vi "AlliGator Highlight Phasor ROI in Original Image v3.vi"(0 "AlliGator IV DVR in":refnum<data-value>, 1 "Image Color Scale Information":T2, 2 "Temp Overlay?":bool, 5 "Source Image Display":T1, 7 "Phasor Plot Image":T1, 9 "Phasor Plot ROI":T3, 11 "Error In":errorcluster, 12 "Overlay Color":u32(colorbox)) -> (4 "AlliGator IV DVR out":refnum<data-value>, 6 "Source Image Display out":T1, 8 "Phasor Plot Image Out":T1, 14 "CPU (s)":dbl, 15 "Error Out":errorcluster)   [LabVIEW 2021, in "AlliGator Source Image.lvlib"]
doc: "Compute and overlays the selected Phasor Plot ROI's pixels in the Source Image."
uses:
  AlliGator Source Image.lvlib
  Internal Variables/AlliGator Internal Variables v2.ctl
  <vilib>/vision/Image Controls.llb/IMAQ Image.ctl
  Internal Variables/AlliGator Gate Image Set.ctl
  Files/AlliGator FLI Dataset Type.ctl
  Files/AlliGator Data Series Type.ctl
  Dual-Channel Datasets/AlliGator Dataset Channel.ctl
  Settings/AlliGator Gate Arithmetic.ctl
  AlliGator Displayed Image.ctl
  Image/Named ROI Description.ctl
  Phasor Graph/AlliGator Decay Metadata v3.ctl
  Decay Analysis/Decay Preprocessing/AlliGator Decay Background Subtraction Info.ctl
  Decay Analysis/Decay Preprocessing/AlliGator Baseline Subtraction Method.ctl
  Graphs/XY Graph/XY Graph Plot Shift Parameters.ctl
  Graphs/XY Graph/XY Graph Plot Shift Method.ctl
  Decay Analysis/Decay Preprocessing/AlliGator Decay Extrapolation Parameters.ctl
  Phasor/Calibration Phasor (m, phi).ctl
  Phasor/Phasor Reference Series.ctl
  Phasor/Phasor Calibration Map v2.ctl
  Phasor/Phasor (g, s).ctl
  Phasor Graph/AlliGator Raw Phasor Plot Data v5.ctl
  Phasor/Phasor Standard Deviation Options.ctl
  Phasor Plot/AlliGator Phasor Multi-Harmonic Data.ctl
  Phasor/Phasor Harmonic Data.ctl
  Decay Fit Parameter Map/AlliGator Decay Fit Options & Parameters v4.ctl
  Fits/IRF(X)PSED/Decay Fit Options v4.ctl
  Fits/Decay Convolution/Decay Model.ctl
  Fits/Residual Type.ctl
  Fits/IRF(X)PSED/Fit Weights Type v2.ctl
  Fits/Non-linear Fitting Method v2.ctl
  Fits/Fit Calculation Method.ctl
  Fits/Non-linear Fitting Algorithm.ctl
  Decay Analysis/Decay Fit/AlliGator Decay Fit Parameter Constraints 2.ctl
  Fits/IRF(X)PSED/Decay Fit Parameters In List.ctl
  Fits/IRF(X)PSED/MLE Baseline Offset Type.ctl
  Decay Analysis/Decay Preprocessing/AlliGator Decay Preprocessing Parameters.ctl
  Fits/IRF(X)PSED/Decay Fit Parameters & Derived Quantities List v2.ctl
  Fits/IRF(X)PSED/Decay Fit Result Constraint.ctl
  Decay Fit Parameter Map/AlliGator Parameter Maps Data.ctl
  Image/Image Color Scale Information.ctl
  Globals, Variables, Constants/AlliGator Variables List.ctl
  Phasor Ratio/AlliGator Phasor Plot Reference Points.ctl
  ROIs/AlliGator ROI Manager Actions.ctl
  Palette/Image Palette Information.ctl
  Image/Image Display Palette Type.ctl
  Settings/AlliGator Settings List.ctl
  9cfa6bdc-d1e0-4e6c-94b8-050a3d16fc11.vi
  Variant/Variant to Data/Variant to Boolean.vi
  <vilib>/vision/NI_Vision_Development_Module.lvlib
  Globals, Variables, Constants/AlliGator Globals, Variables & Constants.lvlib
  Phasor Ratio/AlliGator Phasor Ratio.lvlib
  Error/Error.lvlib
  Settings/AlliGator Settings.lvlib
  Variant/Variant to Data/Variant to Data.lvlib
  Time/Time.lvlib
  ROIs/AlliGator ROIs.lvlib
  Utilities/Utilities.lvlib
  Image/Image.lvlib
  Palette/Palette.lvlib
  Phasor/Phasor.lvlib
  Decay Analysis/Decay Preprocessing/AlliGator Decay Preprocessing.lvlib
  Graphs/XY Graph/XY Graph Add-Ons.lvlib
  Phasor Graph/AlliGator Phasor Graph.lvlib
  Files/AlliGator Files.lvlib
  Phasor Plot/AlliGator Phasor Plot.lvlib
  Internal Variables/AlliGator Internal Variables.lvlib
  Fits/Fits.lvlib
  Decay Analysis/Decay Fit/AlliGator Decay Fit.lvlib
  Dual-Channel Datasets/AlliGator Dual-Channel Datasets.lvlib
  Decay Fit Parameter Map/AlliGator Decay Fit Parameter Map.lvlib
panel:
  in  "Image Color Scale":dbl(ramp)
  # "see the AlliGator License on the block diagram (Ctrl+E or Window:Show Block Diagram)"
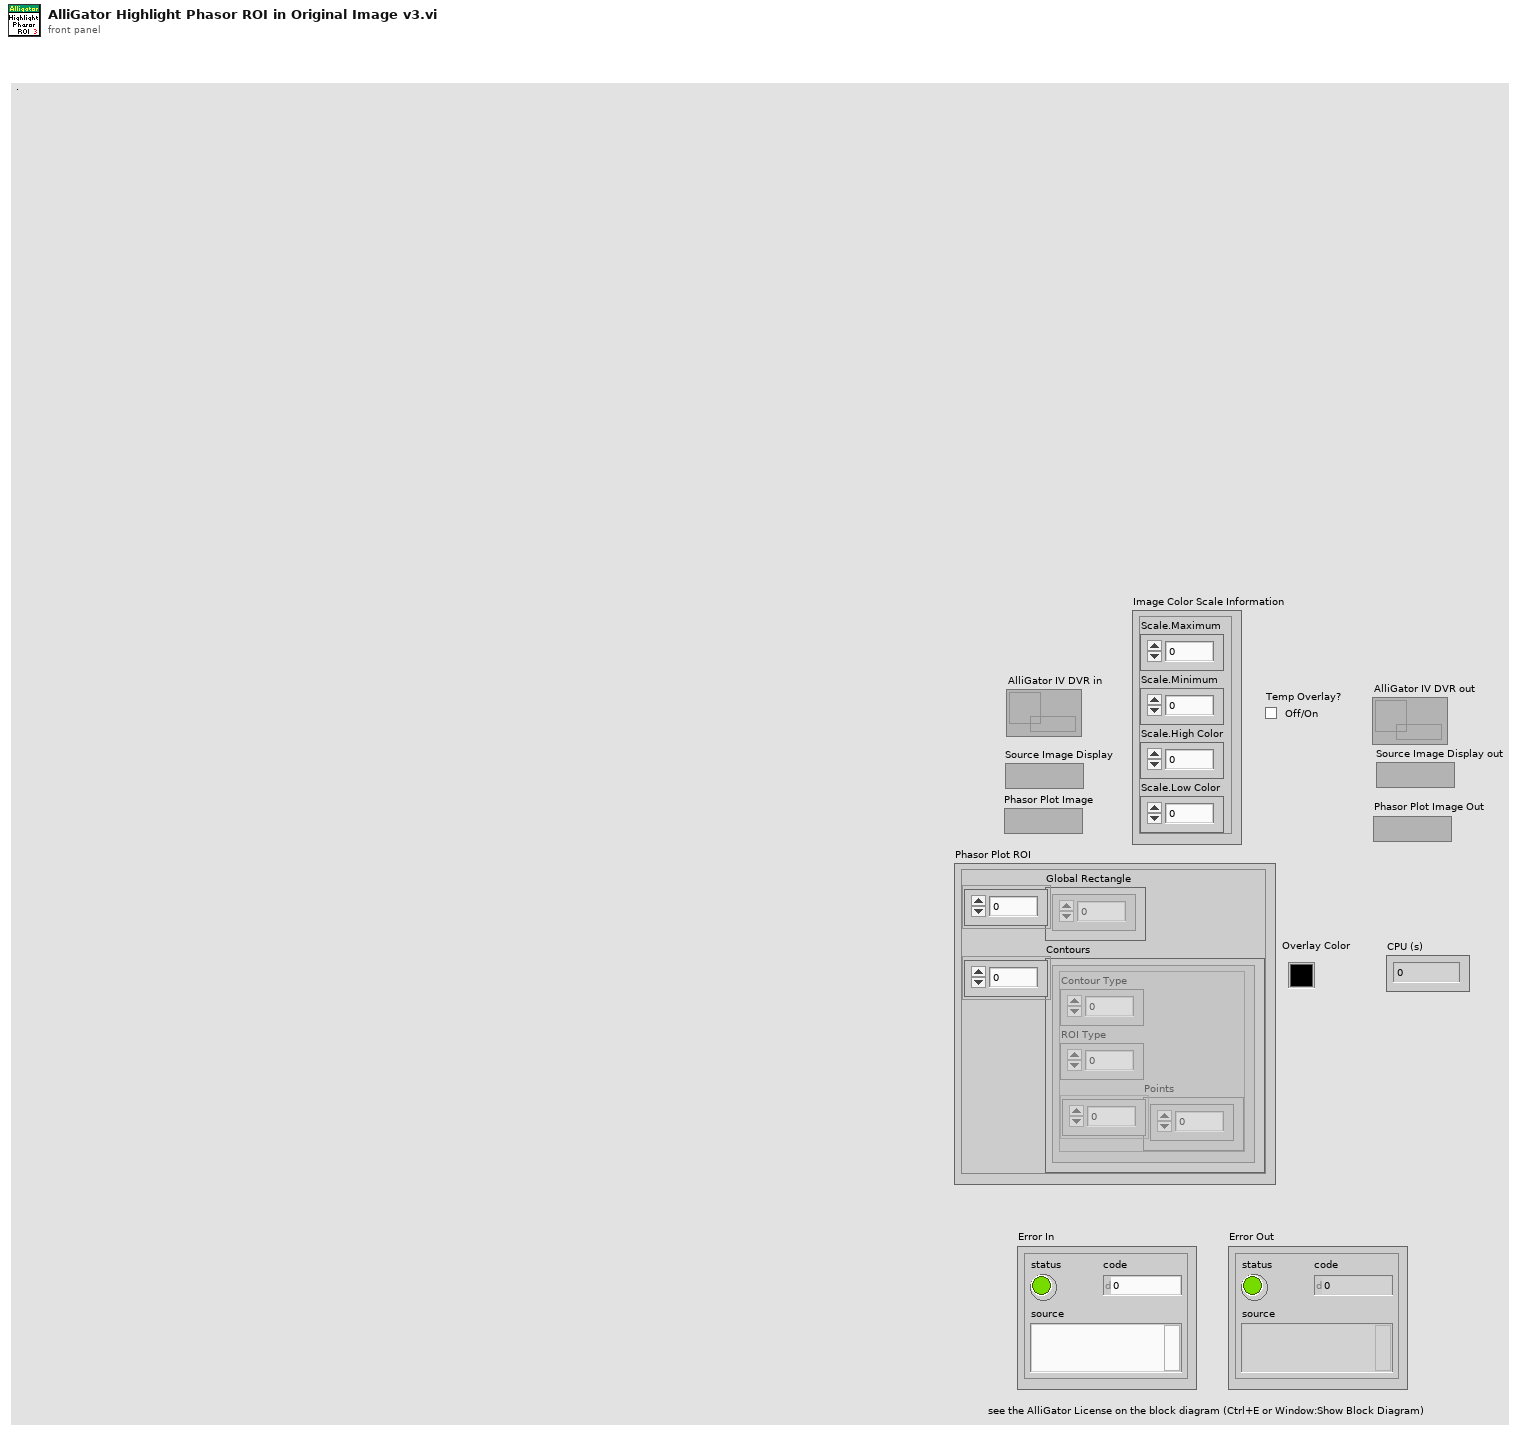
[diagram p1: front panel]
types:
  T1 = typedef "IMAQ Image.ctl" = refnum<image>
  T2 = typedef "Image.lvlib/Image Color Scale Information.ctl" = cluster{"Scale.Maximum":dbl, "Scale.Minimum":dbl, "Scale.High Color":u32, "Scale.Low Color":u32}
  T3 = cluster{"Global Rectangle":i32[], "Contours":cluster{"Contour Type":u32, "ROI Type":u32, "Points":i32[]}[]}
  T4 = typedef "AlliGator Settings.lvlib/AlliGator Settings List.ctl" = enum16{"GUI:Visible Settings Tab", "GUI:Last Run Version", "Source Image:Use Image Histogram for Contrast", "Source Image:Low Count Pixels Rejection Options", "Source Image:High Count Pixels Rejection Options", "Source Image:Use Image Brightness", "Source Image:Blend Overlay with Image Background", "Source Image:Use Fixed ROI Diameter", "Source Image:ROI Diameter", "Source Image:ROI Center Color", "Source Image:Peak Threshold", "Source Image:Intensity Threshold", "Source Image:Image Binning Options", "Source Image:Image Smoothing Options", "Source Image:Image Histogram Active", "Source Image:Invert Binary Mask", "Source Image:Hot Pixel Removal", "Source Image:Overlay Analyzed ROI Center", "Source Image:Auto-Adjust Contrast", "Source Image:Histogram Lower Percentile", "Source Image:Histogram Upper Percentile", "Source Image:Save Source Image", "Source Image:Scale Bar Options", "Source Image:Image Resolution (Pixel Size)", "Source Image:Flatfield Correction", "Source Image:Show Dead Left Columns Correction", "Source Image:Dead Left Columns Correction", "Source Image:Image Pre-Processing Operations Order", "Source Image:Overlay ROI Median", "Source Image:Median Overlay Color", "Data Information:Gate Width", "Data Information:Nanotime Gate Separation", "Data Information:Macrotime Gate Separation", "Data Information:Gate Step", "Data Information:# Gates", "Data Information:Gate Image Exposure", "Data Information:Gate Image Integration", "Data Information:Gates to Skip", "Data Information:Gates to Keep", "Data Information:Define Gates to", "Data Information:Channel Name", "Data Information:Available Channel Names", "Data Information:Channel Arithmetic", "Data Information:Background File Subtraction", "Data Information:Background File", "Data Information:Background Scaling Factor", "Data Information:Background Pile-up Correction", "Data Information:Background Pixel Well Capacity", "Data Information:Laser Period", "Data Information:SYNC Period", "Data Information:Pile-up Correction", "Data Information:Pixel Well Capacity", "Data Information:Dataset Scaling Factor", "Fluorescence Decay_Decay Pre-Processing:Reverse Gates", "Fluorescence Decay_Decay Pre-Processing:Verbose Decay Pre-Processing", "Fluorescence Decay_Decay Pre-Processing:Use Decay Pre-Processing", "Fluorescence Decay_Decay Pre-Processing:Background Subtraction", "Fluorescence Decay_Decay Pre-Processing:Background Definition Range", "Fluorescence Decay_Decay Pre-Processing:Baseline Subtraction Method", "Fluorescence Decay_Decay Pre-Processing:Decay Pre-Processing Operations Order", "Fluorescence Decay_Decay Pre-Processing:Smoothing Parameter", "Fluorescence Decay_Decay Pre-Processing:Shift Decay", "Fluorescence Decay_Decay Pre-Processing:Decay Shift Parameters", "Fluorescence Decay_Decay Pre-Processing:Fold Decay", "Fluorescence Decay_Decay Pre-Processing:# Folds", "Fluorescence Decay_Decay Pre-Processing:1-Normalize Decay", "Fluorescence Decay_Decay Pre-Processing:[0-1]-Normalize Decay", "Fluorescence Decay_Decay Pre-Processing:Smoothen Decay", "Fluorescence Decay_Decay Pre-Processing:Extrapolate Decay", "Fluorescence Decay_Decay Pre-Processing:Use Periodicity", "Fluorescence Decay_Decay Pre-Processing:Use Cursors", "Fluorescence Decay_Decay Pre-Processing:Tail Fraction", "Fluorescence Decay_Decay Pre-Processing:Head Fraction", "Fluorescence Decay_Decay Pre-Processing:Additional Points", "Fluorescence Decay_Decay Pre-Processing:Straighten Decay", "Fluorescence Decay_Decay Pre-Processing:Constant Background", "Fluorescence Decay_Decay Pre-Processing:Pixel-Normalize Decay", "Fluorescence Decay_Advanced Analysis:Extract IRF instead of Decay", "Fluorescence Decay_Advanced Analysis:IRF Extraction Options", "Fluorescence Decay_Advanced Analysis:IRF Optimization Options", "Fluorescence Decay_Advanced Analysis:Square Pulse Options", "Fluorescence Decay_Advanced Analysis:IRF Order", "Fluorescence Decay_Advanced Analysis:IRF Time Constants", "Fluorescence Decay_Advanced Analysis:Wavelet Analysis Options", "Fluorescence Decay_Advanced Analysis:Average Lifetime Options", "Fluorescence Decay_Fit Options:Fit Options", "Fluorescence Decay_Fit Options:Use Legacy Fitting Approach", "Fluorescence Decay_Fit Options:Use Data Information Laser Period", "Fluorescence Decay_Fit Parameters:Displayed Fit Parameters", "Fluorescence Decay_Fit Parameters:Fit Parameter Constraints", "Fluorescence Decay_Fit Parameters:Export Tabulated Results", "Fluorescence Decay_Fit Parameters:MLE Baseline Offset Type", "Fluorescence Decay_Fit Parameters:MLE Baseline Offset", "Fluorescence Decay_Fit Parameters:Guess Parameter Names", "Fluorescence Decay_Fit Parameters:Guess Parameter Values", "Fluorescence Decay_Fit Parameters:Guess Parameters Options", "Fluorescence Decay_Fit Parameters:Optimal Offset Selection Criterion", "Fluorescence Decay_Styles:Show Last Decay Only", "Fluorescence Decay_Styles:Decay Graph Color Array", "Fluorescence Decay:Decay Graph Active", "Fluorescence Decay Statistics:Min Peak Value", "Fluorescence Decay Statistics:Reject Low Decay Peak Pixels", "Fluorescence Decay Statistics:Reject High Decay Peak Pixels", "Fluorescence Decay Statistics:Max Peak Value", "Time Traces:Use File Timestamp", "Time Traces:Time Step", "Time Traces:Use Intensity Correction File", "Time Traces:Intensity Correction File", "Phasor Plot:Phasor Plot Smoothing Options", "Phasor Plot:Phasor Plot Size", "Phasor Plot:Phasor Plot Graphics Options", "Phasor Plot:Cumulative Phasor Plot", "Phasor Plot:Use Phasor Brightness", "Phasor Plot:Blend Overlay with Phasor Background", "Phasor Plot:Save Phasor Plot", "Phasor Plot:Show References", "Phasor Plot:Phasor Ratio Decay Range", "Phasor Plot:Exponential Fading", "Phasor Plot:Phasor Ratio Reference Colors", "Phasor Plot:Reference Radius", "Phasor Plot:Show Color Map Vertices", "Phasor Plot:Phasor Plot Active", "Phasor Plot:Phasor Ratio Color Map Type", "Phasor Plot:Phasor Ratio Color Map", "Phasor Plot:Phasor Ratio Display Range", "Phasor Plot:Selected Image ROI(s)", "Phasor Plot:All Image ROIs", "Phasor Plot:Selected Phasor Plot ROI(s)", "Phasor Plot:All Phasor Plot ROIs", "Phasor Plot:Phasor Ratio Color-Coded Quantity", "Phasor Plot:Store Phasor Harmonics", "Phasor Plot:Draw Reference Segment", "Phasor Plot:User-Defined Quantity", "Phasor Plot:Color Scale High Color", "Phasor Plot:Color Scale Low Color", "Phasor Plot:Intensity-weighted Phasor Plot", "Phasor Graph:Phasor Frequency", "Phasor Graph:Phasor Ratio Type", "Phasor Graph:Pixel-level Phasor Computation", "Phasor Graph:Save Phasor Graph", "Phasor Graph:Phasor Graph Active", "Phasor Graph:Phasor SDV Options", "Phasor Graph:Intensity-weighted Phasor Graph", "Phasor Graph:Define Shortest Lifetime as", "Phasor Calibration:Use Backup Calibration if needed", "Phasor Calibration:Backup Calibration Type", "Phasor Calibration:Calibration Type", "Phasor Calibration:Calibration Lifetime", "Phasor Calibration:Calibration Map Algorithm", "Single-Exponential Phasor Locus (SEPL):Gate Parameters", "Single-Exponential Phasor Locus (SEPL):User-defined Gate", "Single-Exponential Phasor Locus (SEPL):User-defined IRF", "Single-Exponential Phasor Locus (SEPL):Phasor Parameters", "Single-Exponential Phasor Locus (SEPL):Decay & IRF Parameters", "Single-Exponential Phasor Locus (SEPL):Display Parameters", "Lifetime Analysis:Decay Analysis Parameters", "Lifetime Analysis:Lifetime Map Active", "Plugins:Python Settings", "Miscellaneous:Verbose Mode", "Miscellaneous:Beep after Script", "Miscellaneous:Saved Image File Format", "Miscellaneous:Exported Gate Image Settings", "Miscellaneous:Include Loading in Timing", "Miscellaneous:Verbose Settings Mode", "Miscellaneous:Histogram Options", "Miscellaneous:Beep on Error", "Miscellaneous:# Logical Processors Used", "Miscellaneous:ROI Description Max Characters", "Miscellaneous:Verbose Error Mode", "Miscellaneous:Transparent Mask Color"}
  T5 = typedef "Palette.lvlib/Image Palette Information.ctl" = cluster{"Palette Name [# Colors,int?,inv?]":string, "Palette Type":T6, "Palette Colors":u32[], "Interpolate?":bool}
  T6 = typedef "Image.lvlib/Image Display Palette Type.ctl" = u32
  T7 = typedef "AlliGator Globals, Variables & Constants.lvlib/AlliGator Variables List.ctl" = enum16{"---- GUI ----", "GUI:Initialization Status", "GUI:State Indicators Refnum", "GUI:Original AlliGator Menu Items", "GUI:Current Action Loop State", "GUI:Script in progress", "GUI:Playback", "GUI:Loop Playback", "GUI:Search ROI Used", "GUI:Search ROI", "Decay Graph Max Legend Size", "Intensity Graph Max Legend Size", "Decay Statistics Graph Max Legend Size", "Phasor Graph Max Legend Size", "Phasor Ratio Graph Max Legend Size", "Lifetime Graph Max Legend Size", "---- Files ----", "Files:Export Dataset Frames as Individual Files", "Files:Show Batch Export Help Balloons", "Files:Frames in Dataset", "Files:ptu File Frame Start Indices", "Files:Current Frame in Dataset", "Files:Current Frame Timestamp", "Files:Dataset Loaded", "Files:Dataset Metadata", "Files:Dataset Channel", "Files:Dataset Data Description", "Files:Background Dataset Metadata", "Files:Background Dataset Channel", "Files:Background Dataset Data Description", "Files:Background File Subtraction", "Files:Background File Path", "Files:Background File Pile-up Correction", "Files:Background File Pixel Well Capacity", "Files:Background File Scaling Factor", "Files:Current Dataset Load Settings", "Files:Dataset Path", "Files:ICCD-specific Information", "Files:Macrotime Gate Separation", "------ Python Plugins ------", "Python Plugins:Information", "Python Plugins:Python Session", "Python Plugins:Valid Python Session?", "---- Source Image ----", "Source Image:ROIs", "Source Image:Current ROI", "Source Image:ROI Event Refnum", "X_Source Image:Display Range", "X_Source Image:Palette Information", "X_Source Image:Type of Displayed Image", "X_Time Gate Slider", "Source Image:Palette List", "Source Image:Scale", "Source Image:ROI Overlay Color", "Source Image:Overlay to Erase", "Source Image:Is Displayed Image Accumulated", "Source Image:White Light Image Modified", "Source Image:Mask Image Modified", "---- Image Profile Window ----", "Image Profile:Window Event Refnum", "Image Profile:IntensityType", "Image Profile:Intensity Average Type", "Image Profile:Intensity-weighted SDV", "Image Profile:Box Profile Type", "Image Profile:Window Open", "Image Profile:Plotted Fit Parameter", "------ Phasor Graph -------", "Phasor Graph:Show Line", "---- Phasor Plot ---", "Phasor Plot:Parameters Changed", "Phasor Plot:FLI Dataset Modified since last Calculation", "Phasor Harmonics Data", "Selected Phasor Harmonics", "Phasor Harmonic Manager Event Refnum", "Phasor Plot:ROIs", "Phasor Plot:Current ROI", "Phasor Plot:ROI Event Refnum", "Phasor Plot:Image Reference Points", "Phasor Plot:Computed", "Phasor Plot:Palette Information", "Phasor Plot:Palette List", "Phasor Plot:Phasor Ratio Palette Information", "Phasor Plot:Phasor Ratio Palette List", "Phasor Plot:Image Scale", "Phasor Plot:Image Overlay to Erase", "Phasor Plot:Image Elements to Update", "Phasor Plot:Current Calculation Parameters", "Phasor Plot:Current Calibration Options", "Phasor Plot:Reset Cumulated Phasor Plot", "Phasor Plot:Reference 1", "Phasor Plot:Lifetime Reference 1", "Phasor Plot:Reference 1 Frequency", "Phasor Plot:Reference 2", "Phasor Plot:Lifetime Reference 2", "Phasor Plot:Reference 2 Frequency", "---- Decay Analysis ----", "Number of Selected Decays to Fit", "LS Fit Results", "LAR Fit Results", "BS Fit Results", "Last Decay Max - Min", "Best Fit Parameters", "Best Fit Parameter Names", "Actual Size X", "Actual Size Y", "Binning X", "Binning Y", "Actual # Gates", "Dataset Number", "Gates to...", "Gates Skipped", "Gates to keep", "Gate Step", "Gate Separation", "Reversed Gates", "Pile-up Correction", "Pixel Well Capacity", "Background Subtracted", "Background Subtraction Method", "Background Definition Range", "Background File (deprecated)", "Number of Dataset Accumulated", "Array of Accumulated Dataset Paths", "Do Averaged Datasets", "Destination File Path", "Process Plot Target", "Use 1/D as Phasor Frequency", "---- Decay Fit Parameter Map -----", "Decay Fit Parameter Map:Palette Information", "Decay Fit Parameter Map:Palette List", "Decay Fit Parameter Map:X Resolution", "Decay Fit Parameter Map:Y Resolution", "Decay Fit Parameter Map:Use Decay Fit Result Constraints", "Decay Fit Parameter Map:Decay Fit Result Constraints", "Decay Fit Parameter Map:Decay Fit Result Constraints Applied", "---- Parameter Map ----", "Parameter Map:Palette Information", "Parameter Map:Palette List", "------- Local Decay Window ---------", "Local Decay Graph Window:Event Refnum", "Local Decay Graph Window:Use normalized IRF for convolution", "----- Miscellaneous ----", "Misc:Skippable Dialog Windows Status"}
  T8 = typedef "AlliGator ROIs.lvlib/AlliGator ROI Manager Actions.ctl" = enum16{"Undefined", "Delete Current ROI", "Delete All Unselected ROIs", "Delete Multiple ROIs", "Delete All ROIs", "Swap ROIs", "Insert ROI", "Update Current ROI Descriptor", "Rename Current ROI", "Store New ROI", "Store Multiple ROIs", "Select Next ROI", "Select Previous ROI", "Find Selected ROI", "Show All ROIs", "Update ROI Manager Window", "Merge All ROIs", "Unmerge ROI", "Set Selected ROI by ID"}
  T9 = typedef "AlliGator Phasor Ratio.lvlib/AlliGator Phasor Plot Reference Points.ctl" = cluster{"O_h":dbl, "O_v":dbl, "1_h":dbl, "1_v":dbl}
  T10 = typedef "AlliGator Internal Variables.lvlib/AlliGator Internal Variables v2.ctl" = cluster{"----------------------------- Images -----------------------------":u8, "Displayed Image":T1, "White Light Image":T1, "Mask Image":T1, "ROI Mask Image":T1, "Current Dataset Images 1":T11, "Background Dataset Images 1":T11, "Current Dataset Images 2":T11, "Background Dataset Images 2":T11, "Current Dataset Arithmetic Images":T11, "Accumulated Dataset Images 1":T11, "Accumulated Dataset Images 2":T11, "Accumulated Dataset Arithmetic Images":T11, "----------------------------- File Paths -----------------------------":u8, "Phasor Plot Image":T1, "Decay Fit Parameter Map Image":T1, "Parameter Map Image":T1, "Single Data Point Path":path, "White Light Image Path":path, "Mask Image Path":path, "Time-Series Folder":path, "[Time-Series Paths]":path[], "----------------------------- FLI Dataset -----------------------------":u8, "Current Dataset":i32, "Single Dataset Type":T12, "Current Folder":string, "AlliGator Data Series Type":T13, "# Datasets":i32, "Dual-Channel Dataset":bool, "Selected Channel Name":string, "Dataset Channel":T14, "Channel Arithmetic":T15, "Dual-Channel Background Dataset":bool, "Background Channel":T14, "Dual-Channel Accumulated Dataset":bool, "Start Time":dbl, "[Time-Series Timestamps]":dbl[], "[Intensity Corrections]":dbl[], "Time Series Script":bool, "Type of Displayed Image":T16, "Gate Image Slide":u16, "# Gates":i32, "ROIs":T17[], "----------------------------- Decays -----------------------------":u8, "ROI Decay":cluster{"t Array":dbl[], "I Array":dbl[]}, "Valid Decay":bool, "Decay  Metadata":T19, "Reference Decay Plot Name":string, "Reference Decay":cluster{"t Array":dbl[], "I Array":dbl[]}, "Decay Shift Plot":cluster{"Time Stamps":dbl[], "Decay Shifts":dbl[]}, "[Decays Max Values]":sgl[], "[Decays Min Values]":sgl[], "----------------------------- Calibration -----------------------------":u8, "Calibration Phasor":T25, "Calibration Phasor Series":T26, "Phasor Calibration Map":T27, "Calibration Map MD5 Digest":string, "----------------------------- Phasor Graph -----------------------------":u8, "Last Raw Phasor":T28, "Last Calibrated Phasor":T28, "Last Calibrated Phasor SDV":T28, "Phasor Graph:Phasor Plot":cluster{"g Array":dbl[], "s Array":dbl[]}, "Phasor Graph:Phasor SDV Plot":cluster{"g Array":dbl[], "s Array":dbl[]}, "[Phasor Graph:Raw Phasor Plots]":T29[], "Phasor Plot locked to Ref 1":i32, "[Phasor Plot(s) locked to Ref 1]":i32[], "[Phasor Plot(s) locked to Ref 2]":i32[], "[Pixel Phasors]":T28[], "----------------------------- Phasor Plot -----------------------------":u8, "[[Sum Image]]":dbl[][], "[[CSG Phasors]]":csg[][], "[[Valid Pixel?]]":bool[][], "[[Phasor Ratios]]":dbl[][], "[[Average Lifetimes]]":dbl[][], "Amplitude Weighted Average Lifetime":bool, "I/m/phi Dataset":cluster{"I/m/phi Dataset?":bool, "Base Frequency":dbl[unit], "Harmonic Orders":u8[]}, "Multi Phasor Plot Data":T31, "----------------------------- Decay Fit Parameter Map -----------------------------":u8, "Decay Fit Options & Parameters":T33, "Fit Options: Decay Preprocessing Parameters":T44, "Fit Options: Reference Decay":cluster{"t Array":dbl[], "I Array":dbl[]}, "Is Full Image Parameters Map":bool, "Is Single-Pixels Parameters Map":bool, "NLSF Parameters Map X Resolution":i32, "NLSF Parameters Map Y Resolution":i32, "[Single Decay Fit Parameters]":dbl[], "Fit Model":T35, "[[Multiple Decays Fit Parameters]]":dbl[][], "[[Multiple Decays Fit Parameter SDVs]]":dbl[][], "[[IRFs]]":dbl[][], "[ROI Descriptors]":T18[], "IRF Array Time Axis":dbl[], "Decay Array Time Axis":dbl[], "[Decay Fit Parameter Names]":T45[], "[Decay Sum]":dbl[], "Array of Decay Fit Result Constraints":T46[], "Selected ROIs Array":bool[], "----------------------------- Parameter Maps -----------------------------":u8, "[Map Set Names]":string[], "[Parameter Maps]":T47[], "[[User-defined Quantities]]":dbl[][], "User-defined Quantity":string}
  T11 = typedef "AlliGator Internal Variables.lvlib/AlliGator Gate Image Set.ctl" = cluster{"SGL Gate Images":T1[], "SGL Sum Image":T1, "SGL Max Image":T1, "SGL Min Image":T1}
  T12 = typedef "AlliGator Files.lvlib/AlliGator FLI Dataset Type.ctl" = enum16{"HDF5 FLI Dataset", "Gate Image Folder", ".sdt FLI Dataset (Becker & Hickl)", ".ptu FLI Dataset (PicoQuant)", "SS1 FLI Dataset", "SS2 FLI Dataset", "I/m/phi Dataset", ".bin FLI Dataset (PicoQuant Binned)", ".bin FLI Dataset (Piccolo Binned)", ".mat FLI Dataset"}
  T13 = typedef "AlliGator Files.lvlib/AlliGator Data Series Type.ctl" = enum16{"Not a Supported Series", "Gate Images Folder Series", "SwissSPAD 2 Dataset Series", "B&H FLI Dataset Series", "PicoQuant PTU FLI Dataset Series", "PicoQuant BIN FLI Dataset Series", "Piccolo hist BIN FLI Dataset Series", "HDF5 FLI Dataset Series"}
  T14 = typedef "AlliGator Dual-Channel Datasets.lvlib/AlliGator Dataset Channel.ctl" = enum16{"G2", "INT"}
  T15 = typedef "AlliGator Settings.lvlib/AlliGator Gate Arithmetic.ctl" = enum16{"None", "INT-G2", "G2/INT*<INT>", "(1 - G2/INT)*<INT>"}
  T16 = typedef "AlliGator Source Image.lvlib/AlliGator Displayed Image.ctl" = enum16{"Single Gate", "Sum of All Gates", "Max of All Gates", "Min of All Gates", "-", "White Ligth Image", "Mask Image"}
  T17 = typedef "Image.lvlib/Named ROI Description.ctl" = cluster{"ROI Descriptor":T18, "ROI Name":string, "Overlay Color":u32}
  T18 = typedef "ROI Descriptor" = cluster{"Global Rectangle":i32[], "Contours":cluster{"ID":enum32{"External", "Internal"}, "Type":u32, "Coordinates":i32[]}[]}
  T19 = typedef "AlliGator Phasor Graph.lvlib/AlliGator Decay Metadata v3.ctl" = cluster{"ROI Descriptor":T18, "ROI Center":cluster{"X":i32, "Y":i32}, "Decay Background Subtraction Info":T20, "Decay Reverted":bool, "Decay Smoothened":bool, "Decay Straightened":bool, "Fitted Tau (Decay Straightening)":dbl, "Decay Shift Parameters":T22, "Decay Shifted":bool, "Decay Extrapolated":bool, "Decay Extrapolation Parameters":T24, "Decay Normalized":bool, "Fold Decay":bool, "# Folds":u32}
  T20 = typedef "AlliGator Decay Preprocessing.lvlib/AlliGator Decay Background Subtraction Info.ctl" = cluster{"Laser Period":dbl[unit], "Gate Duration":dbl[unit], "Baseline Subtraction Method":T21, "Background Definition Range":cluster{"Min Gate":dbl[unit], "Max Gate":dbl[unit]}, "Total Intensity w/o Bkgd Subtraction":dbl, "Bkgd-subtracted Intensity (exp)":dbl, "# Data Points":i32, "Background/Gate":dbl, "Fitted Lifetime":dbl[unit], "Bkgd-subtracted Intensity (theo)":dbl}
  T21 = typedef "AlliGator Decay Preprocessing.lvlib/AlliGator Baseline Subtraction Method.ctl" = enum16{"Mean", "Min", "Square Gated Single-Exponential", "File", "Constant"}
  T22 = typedef "XY Graph Add-Ons.lvlib/XY Graph Plot Shift Parameters.ctl" = cluster{"Type":T23, "Shift":dbl[unit], "Threshold":dbl, "Rotate":bool}
  T23 = typedef "XY Graph Add-Ons.lvlib/XY Graph Plot Shift Method.ctl" = enum16{"Default", "CFD", "Threshold", "Cross-Correlation"}
  T24 = typedef "AlliGator Decay Preprocessing.lvlib/AlliGator Decay Extrapolation Parameters.ctl" = cluster{"Additional Points":u32, "Head Fraction":dbl, "Fitted Tau":dbl, "Use Periodicity":bool, "Use Cursors":bool, "Tail Fraction":dbl}
  T25 = typedef "Phasor.lvlib/Calibration Phasor (m, phi).ctl" = cluster{"m":dbl, "phi":dbl, "Phasor Frequency":dbl[unit], "Reference Lifetime":dbl[unit]}
  T26 = typedef "Phasor.lvlib/Phasor Reference Series.ctl" = cluster{"m Array":dbl[], "phi Array":dbl[], "Phasor Frequency":dbl[unit], "Calibration Lifetime":dbl[unit]}
  T27 = typedef "Phasor.lvlib/Phasor Calibration Map v2.ctl" = cluster{"Phasor Frequency":dbl[unit], "Calibration Lifetime":dbl[unit], "ROI Centers":cluster{"X":i32, "Y":i32}[], "ROI Descriptors":T18[], "Map Resolution X":i32, "Map Resolution Y":i32, "z Array":cdb[]}
  T28 = typedef "Phasor.lvlib/Phasor (g, s).ctl" = cluster{"g":dbl, "s":dbl}
  T29 = typedef "AlliGator Phasor Graph.lvlib/AlliGator Raw Phasor Plot Data v5.ctl" = cluster{"Phasor Plot Name":string, "Raw Phasor Plot":T28[], "Phasor Frequency":dbl[unit], "[Decay Metadata]":T19[], "Raw Phasor Plot SDV":T28[], "Phasor SDV Options":T30, "[Calibration Phasor]":T25[], "Intensity Array":dbl[]}
  T30 = typedef "Phasor.lvlib/Phasor Standard Deviation Options.ctl" = cluster{"Compute Estimated SDV":bool, "# Replicas":u32, "Use Estimated Average Phasor":bool}
  T31 = typedef "AlliGator Phasor Plot.lvlib/AlliGator Phasor Multi-Harmonic Data.ctl" = cluster{"Base Frequency":dbl[unit], "# Harmonics":u8, "Harmonic Orders":u8[], "Phasor Plot Settings Checksum":u64, "Phasor Harmonic Data Array":T32[]}
  T32 = typedef "Phasor.lvlib/Phasor Harmonic Data.ctl" = cluster{"Phasor Harmonic Name":string, "Phasor Plot Settings Checksum":u64, "Phasor Frequency":dbl[unit], "Base Frequency":dbl[unit], "Harmonic Order":u8, "Phasor Plot Parameters":string, "Phasor Array [[CSG]]":csg[][], "Dataset File Path":path}
  T33 = typedef "AlliGator Decay Fit Parameter Map.lvlib/AlliGator Decay Fit Options & Parameters v4.ctl" = cluster{"SYNC Period":dbl[unit], "Fit Options":T34, "Fit Parameter Constraints":T41[], "MLE Baseline Offset":dbl, "MLE Baseline Offset Type":T43}
  T34 = typedef "Fits.lvlib/Decay Fit Options v4.ctl" = cluster{"Show Fit Residuals":bool, "Fit Model":T35, "Residual Type":T36, "Max Decay Percentile":dbl, "Min Decay Percentile":dbl, "Show Full Decay":bool, "Weights":T37, "Fitting Method":T38, "Compute Parameter Uncertainties":bool, "Periodic Boundaries":bool, "Model Calculation":T39, "Period":dbl[unit], "Termination Criteria":cluster{"Max Iterations":i32, "Max Function Calls":i32, "Max Time":dbl[unit], "Function Tolerance":dbl, "Parameter Tolerance":dbl, "Gradient Tolerance":dbl, "Min Lambda":dbl, "Max Lambda":dbl, "Initial Tick Count":u32}, "Offset Resolution":dbl[unit], "Use Local IRF":bool, "Fitting Algorithm":T40, "Show Confidence Interval ":bool, "Confidence Level":dbl}
  T35 = typedef "Fits.lvlib/Decay Model.ctl" = enum16{"1-Exponential", "2-Exponentials"}
  T36 = typedef "Fits.lvlib/Residual Type.ctl" = enum16{"Standard", "Normalized", "Reduced"}
  T37 = typedef "Fits.lvlib/Fit Weights Type v2.ctl" = enum16{"Unweighted", "1/Variance (Neyman)", "1/Variance (Pearson)", "Best of All"}
  T38 = typedef "Fits.lvlib/Non-linear Fitting Method v2.ctl" = enum16{"Least Square", "Least Absolute Residual", "Bisquare", "MLE", "-", "Best of All"}
  T39 = typedef "Fits.lvlib/Fit Calculation Method.ctl" = enum16{"Simulation", "Convolution", "Integration"}
  T40 = typedef "Fits.lvlib/Non-linear Fitting Algorithm.ctl" = enum16{"Levenberg-Marquardt", "Trust-Region Dogleg"}
  T41 = typedef "AlliGator Decay Fit.lvlib/AlliGator Decay Fit Parameter Constraints 2.ctl" = cluster{"Fit Parameter":T42, "Min Value":dbl, "Max Value":dbl, "Global":bool, "Used":bool}
  T42 = typedef "Fits.lvlib/Decay Fit Parameters In List.ctl" = enum16{"Offset", "Baseline", "A_1", "tau_1", "A_2", "tau_2"}
  T43 = typedef "Fits.lvlib/MLE Baseline Offset Type.ctl" = enum32{"Absolute", "Percentage"}
  T44 = typedef "AlliGator Decay Preprocessing.lvlib/AlliGator Decay Preprocessing Parameters.ctl" = cluster{"Background Subtraction":bool, "Straighten Decay":bool, "Reverse Gates":bool, "1-Normalized Decay":bool, "Smoothen Decay":bool, "Smoothing Parameter":dbl, "Shift Decay":bool, "Decay Shift Parameters":T22, "Extrapolate Decay":bool, "Additional Points":u32, "Head Fraction":dbl, "Pixel-Normalize Decay":bool, "Use Periodicity":bool, "Use Cursors":bool, "Tail Fraction":dbl, "Use Decay Pre-Processing":bool, "Fold Decay":bool, "# Folds":u32, "[0-1]-Normalized Decay":bool}
  T45 = typedef "Fits.lvlib/Decay Fit Parameters & Derived Quantities List v2.ctl" = enum16{"Offset", "Baseline", "A_1", "tau_1", "A_2", "tau_2", "<tau>_a", "f1_a", "f2_a", "<tau>_i", "f1_i", "f2_i", "-", "R^2", "Chi^2"}
  T46 = typedef "Fits.lvlib/Decay Fit Result Constraint.ctl" = cluster{"Fit Parameter":enum16{"Offset", "Baseline", "A_1", "tau_1", "A_2", "tau_2", "<tau>_a", "f1_a", "f2_a", "<tau>_i", "f1_i", "f2_i", "-", "R^2", "Chi^2", "Max Relative Residual", "<Residual ACF>", "Residual ACF SDV", "tau_2/tau_1"}, "Min Value":dbl, "Max Value":dbl, "Use Constraint":bool}
  T47 = typedef "AlliGator Decay Fit Parameter Map.lvlib/AlliGator Parameter Maps Data.ctl" = cluster{"Map Set Name":string, "[Parameter Names]":string[], "[[Parameters]]":dbl[][], "[[Parameter SDVs]]":dbl[][], "Decay Array Time Axis":dbl[], "[[IRFs]]":dbl[][], "IRF Array Time Axis":dbl[], "X Resolution":i32, "Y Resolution":i32, "Intensity Array":dbl[]}
  T48 = typedef "Image Type" = u32
  T49 = cluster{"Red (or Hue) value":u8, "Green (or Sat) value":u8, "Blue (or Light or Val) value":u8}
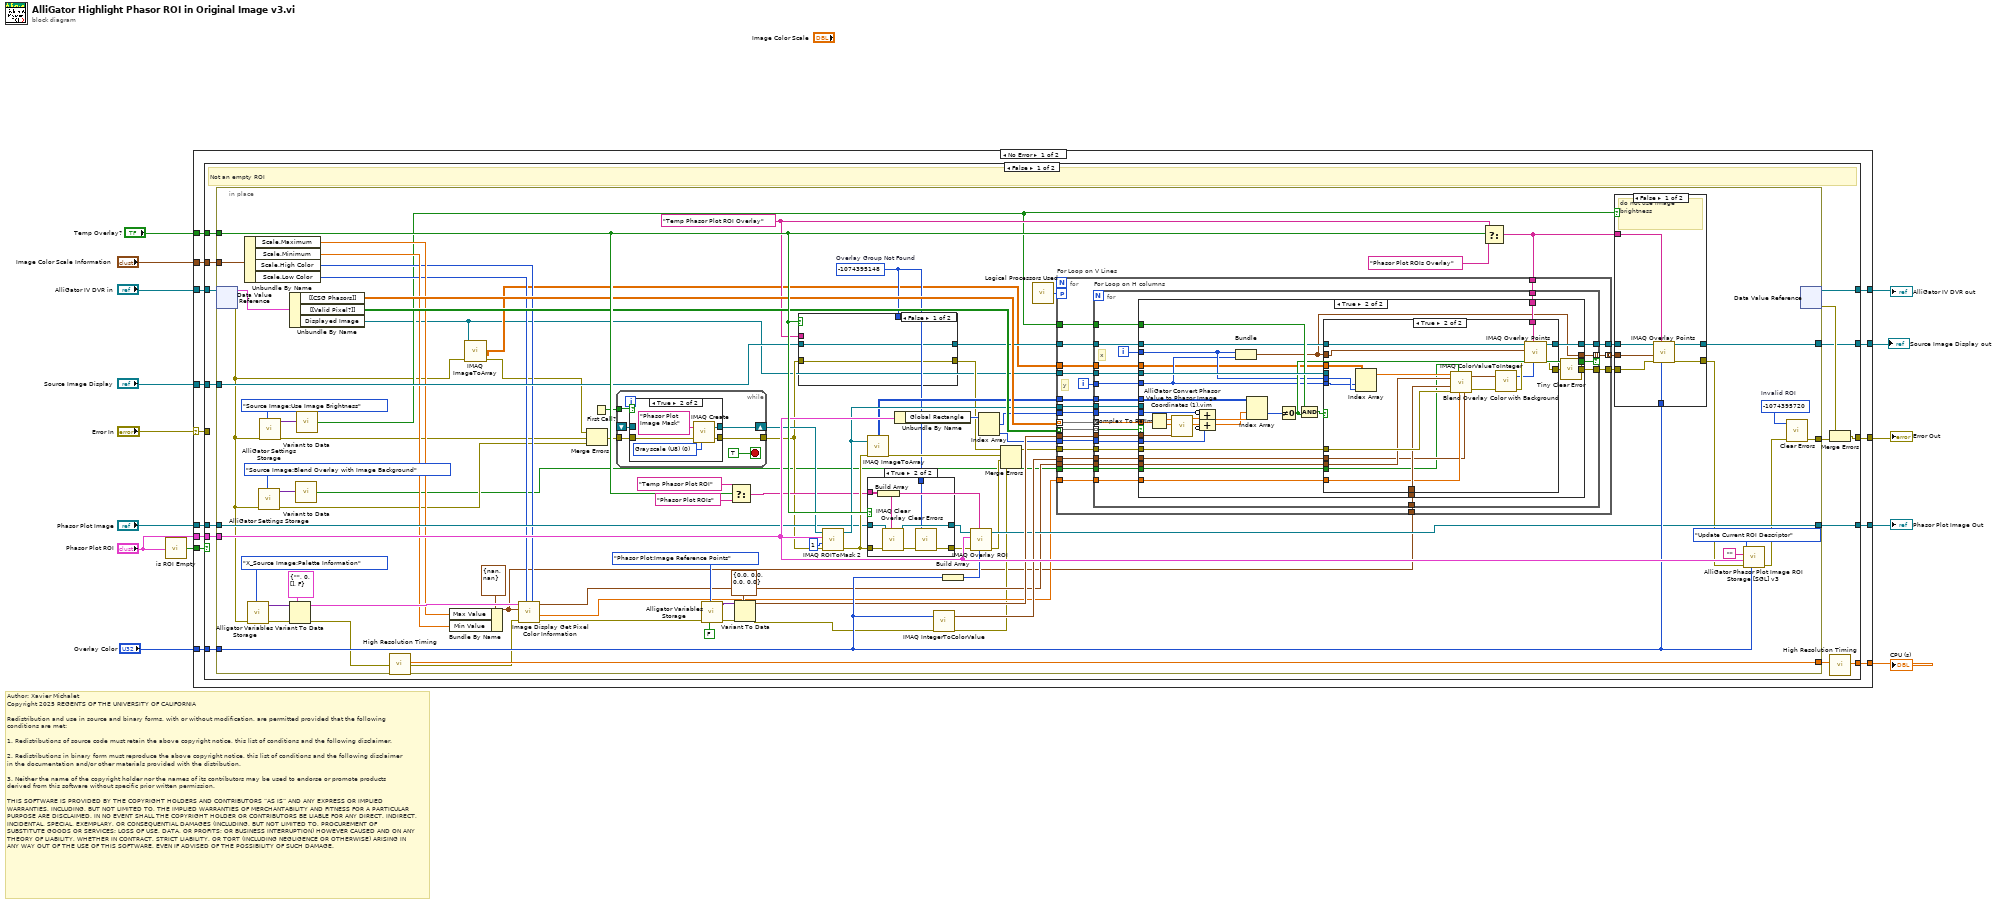
[diagram p0: block diagram]
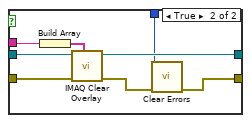
[diagram p6: hidden frame]
diagram:
  # "Author: Xavier Michalet\nCopyright 2025 REGENTS OF THE UNIVERSITY OF CALIFORNIA\n\nRedistribution and use in source and binary forms, with or without modification, are permitted provided that the following conditions are met:\n\n1. Redistributions of source code must retain the above copyright notice, this list of conditions and the following disclaimer.\n\n2. Redistributions in binary form must reproduce the above copyright notice, this list of conditions and the following disclaimer in the documentation and/or other materials provided with the distribution.\n\n3. Neither the name of the copyright holder nor the names of its contributors may be used to endorse or promote products derived from this software without specific prior written permission.\n\nTHIS SOFTWARE IS PROVIDED BY THE COPYRIGHT HOLDERS AND CONTRIBUTORS “AS IS” AND ANY EXPRESS OR IMPLIED WARRANTIES, INCLUDING, BUT NOT LIMITED TO, THE IMPLIED WARRANTIES OF MERCHANTABILITY AND FITNESS FOR A PARTICULAR PURPOSE ARE DISCLAIMED. IN NO EVENT SHALL THE COPYRIGHT HOLDER OR CONTRIBUTORS BE LIABLE FOR ANY DIRECT, INDIRECT, INCIDENTAL, SPECIAL, EXEMPLARY, OR CONSEQUENTIAL DAMAGES (INCLUDING, BUT NOT LIMITED TO, PROCUREMENT OF SUBSTITUTE GOODS OR SERVICES; LOSS OF USE, DATA, OR PROFITS; OR BUSINESS INTERRUPTION) HOWEVER CAUSED AND ON ANY THEORY OF LIABILITY, WHETHER IN CONTRACT, STRICT LIABILITY, OR TORT (INCLUDING NEGLIGENCE OR OTHERWISE) ARISING IN ANY WAY OUT OF THE USE OF THIS SOFTWARE, EVEN IF ADVISED OF THE POSSIBILITY OF SUCH DAMAGE."
  n1 = call "is ROI Empty.vi"("Current ROI Descriptor"="Phasor Plot ROI") -> ("Empty ROI?"=w9:bool)  [unwired: 8 in]
  n2 = case shown="No Error" "Error In" {
    selector: "Error In" -> [w15 w276]
    tunnel: "Overlay Color" -> [w28 _]
    tunnel: "AlliGator IV DVR in" -> [w27 w278]
    tunnel: [w26 w278] -> w12
    tunnel: [w25 w276] -> w11
    tunnel: "Temp Overlay?" -> [w24 _]
    tunnel: w9 -> [w23 _]
    tunnel: [w22 _] -> w8
    tunnel: "Phasor Plot ROI" -> [w21 _]
    tunnel: "Phasor Plot Image" -> [w20 w275]
    tunnel: [w19 w275] -> w5
    tunnel: "Source Image Display" -> [w18 w277]
    tunnel: [w17 w277] -> w3
    tunnel: "Image Color Scale Information" -> [w16 _]
    frame No Error {
      n3 = case shown="False" w23 {
        tunnel: w28 -> [w42 _]
        tunnel: w27 -> [w41 w274]
        tunnel: [w40 w274] -> w26
        tunnel: [w39 w271] -> w25
        tunnel: w24 -> [w37 _]
        tunnel: w20 -> [w36 w272]
        tunnel: w21 -> [w35 _]
        tunnel: [w33 _] -> w22
        tunnel: [w32 w272] -> w19
        tunnel: w18 -> [w31 w273]
        tunnel: [w30 w273] -> w17
        tunnel: w16 -> [w29 _]
        tunnel: w15 -> [_ w271]
        frame False {
          # "Not an empty ROI"
          n4 = in-place {
            in-place-border: w36 -> [w83]
            in-place-border: [w128] -> w43
            in-place-border: w42 -> [w120]
            in-place-border: [w127] -> w34
            in-place-border: w37 -> [w125]
            in-place-border: w35 -> [w124]
            in-place-border: [w82] -> w32
            in-place-border: w31 -> [w71]
            in-place-border: [w80] -> w30
            in-place-border: w29 -> [w62]
            w84 = -1074395148  # Overlay Group Not Found
            w92 = "Temp Phasor Plot ROI Overlay" ("Group")
            w121 = -1074395720  # Invalid ROI
            n5 = in-place-dvr #1(w41) -> (w126:T10, w51:errorcluster)
            n6 = Unbundle By Name(w62) -> ("Scale.Maximum"=w61:dbl, "Scale.Minimum"=w60:dbl, "Scale.High Color"=w59:u32, "Scale.Low Color"=w58:u32)
            n7 = call "Alligator Variables Storage.vi"("AlliGator Variable"=AlliGator_Variables_List."X_Source Image:Palette Information" ("Alligator Variable"), "Error In"=w51) -> ("Error Out"=w77:errorcluster, "Data out"=w76:variant)  [unwired: 7 in, 1 out]
            n8 = call "AlliGator Settings Storage.vi"("AlliGator Settings List"=AlliGator_Settings_List."Source Image:Blend Overlay with Image Background", "Error In"=w51) -> ("Error Out"=w49:errorcluster, "Variant Data out"=w53:variant)  [unwired: 8 in]
            n9 = call "AlliGator Settings Storage.vi"("AlliGator Settings List"=AlliGator_Settings_List."Source Image:Use Image Brightness", "Error In"=w51) -> ("Error Out"=w55:errorcluster, "Variant Data out"=w57:variant)  [unwired: 8 in]
            n10 = Variant To Data(error in=w77, type=T5 {"Palette Name [# Colors,int?,inv?]"="", "Palette Type"=0, "Palette Colors"=[], "Interpolate?"=FALSE} ("Image Display Palette Information"), Variant=w76) -> (data=w74:T5, error out=w68:errorcluster)
            n11 = Unbundle By Name(w126) -> ("[[CSG Phasors]]"=w122:csg[][], "[[Valid Pixel?]]"=w123:bool[][], "Displayed Image"=w45:T1)
            n12 = call-poly "Variant to Data.vi"("Variant"=w53) -> ("Value"=w47:bool)  [unwired: 8 in]
            n13 = call-poly "Variant to Data.vi"("Variant"=w57) -> ("Value"=w54:bool)  [unwired: 8 in]
            n14 = call "High Resolution Timing.vi"("Error In"=w68) -> ("elapsed (relative) seconds"=w127:dbl, "Error Out"=w67:errorcluster)  [unwired: 16 in, 1 out]
            n15 = Bundle By Name(cluster=cluster{"Min Value":sgl, "Max Value":sgl} {"Min Value"=nan, "Max Value"=nan} ("Image Display Range"), "Max Value"=w61, "Min Value"=w60) -> (w44:cluster{"Min Value":sgl, "Max Value":sgl})
            n16 = call "IMAQ ImageToArray"("error in (no error)"=w51, "Image"=w45) -> ("Image Pixels (Float)"=w46:sgl[][], "error out"=w48:errorcluster)  [unwired: 2 in, 3 out]
            n17 = call "Image Display Get Pixel Color Information.vi"("Image High Color"=w59, "Image Low Color"=w58, "Error In"=w67, "Image Display Range"=w44, "Image Display Palette Information"=w74) -> ("Error Out"=w72:errorcluster, "Image Scale Factor (256 colors)"=w69:sgl, "1D Color Array"=w70:cluster{"Red":u8, "Green":u8, "Blue":u8}[])  [unwired: 3 in, 1 out]
            n18 = Merge Errors(w48, w55, w49) -> (w50:errorcluster)
            n19 = First Call?() -> (First Call?: T/F=w118:bool)
            n20 = while {
              tunnel: w118 -> [w263]
              tunnel: w50 -> [w262]
              shift-right: [w261] -> w88
              shift-left: _ -> [w259]
              tunnel: [w258] -> w79
              stop <- TRUE stop-if-true
              n21 = case shown="True" w263 {
                tunnel: w262 -> [w264 w269]
                tunnel: [w265 w268] -> w261
                tunnel: w259 -> [w265 _]
                tunnel: [w264 w267] -> w258
                frame False {
                }
                frame True {
                  w266 = T48 0 items=["Grayscale (U8)", "Grayscale (I16)", "Grayscale (SGL)", "Complex (CSG)", "RGB (U32)", "HSL (U32)", "RGB (U64)", "Grayscale (U16)"] ("Image Type")
                  n22 = call "IMAQ Create"("Image Name"="Phasor Plot Image Mask", "Image Type"=w266, "error in (no error)"=w269) -> ("New Image"=w268:T1, "error out"=w267:errorcluster)  [unwired: 2 in]
                }
              }
            }
            n23 = call "Alligator Variables Storage.vi"("Get(F)/Set"=FALSE, "AlliGator Variable"=AlliGator_Variables_List."Phasor Plot:Image Reference Points" ("Alligator Variable"), "Error In"=w72) -> ("Error Out"=w113:errorcluster, "Data out"=w115:variant)  [unwired: 6 in, 1 out]
            n24 = Select(t="Temp Phasor Plot ROI" ("Group"), s=w125, f="Phasor Plot ROIs" ("Group")) -> (s? t:f=w85:string)
            n25 = Variant To Data(error in=w113, type=T9 {"O_h"=0.0, "O_v"=0.0, "1_h"=0.0, "1_v"=0.0} ("Phasor Plot Reference Points"), Variant=w115) -> (data=w112:T9, error out=w66:errorcluster)
            n26 = case shown="False" w125 {
              tunnel: w71 -> [w249 w257]
              tunnel: [w249 w256] -> w94
              tunnel: w79 -> [w248 w253]
              tunnel: [w248 w251] -> w93
              tunnel: w92 -> [_ w255]
              tunnel: w84 -> [_ w250]
              frame False {
              }
              frame True {
                n27 = Build Array(w255) -> (w254:string[])
                n28 = call "IMAQ Clear Overlay"("Groups"=w254, "error in (no error)"=w253, "Image"=w257) -> ("error out"=w252:errorcluster, "Image Out"=w256:T1)  [unwired: 7 in]
                n29 = call <vilib>:"Clear Errors.vi"("error in (no error)"=w252, "specific error code to clear (0: all)"=w250) -> ("error out"=w251:errorcluster)  [unwired: 4 in, 1 out]
              }
            }
            n30 = call "IMAQ ROIToMask 2"("error in (no error)"=w79, "Filling Value (255)"=1, "ROI Descriptor"=w124, "Image"=w88) -> ("error out"=w90:errorcluster, "Image Out"=w103:T1)  [unwired: 5 in, 1 out]
            n31 = call "IMAQ ImageToArray"("error in (no error)"=w90, "Image"=w103) -> ("error out"=w101:errorcluster, "Image Pixels (U8)"=w102:u8[][])  [unwired: 2 in, 3 out]
            n32 = case shown="True" w125 {
              tunnel: w83 -> [w239 w245]
              tunnel: [w239 w244] -> w91
              tunnel: w90 -> [w238 w243]
              tunnel: [w238 w241] -> w89
              tunnel: w85 -> [_ w246]
              tunnel: w84 -> [_ w240]
              frame False {
              }
              frame True {
                n33 = Build Array(w246) -> (w247:string[])
                n34 = call "IMAQ Clear Overlay"("Groups"=w247, "error in (no error)"=w243, "Image"=w245) -> ("error out"=w242:errorcluster, "Image Out"=w244:T1)  [unwired: 7 in]
                n35 = call <vilib>:"Clear Errors.vi"("error in (no error)"=w242, "specific error code to clear (0: all)"=w240) -> ("error out"=w241:errorcluster)  [unwired: 4 in, 1 out]
              }
            }
            n36 = Unbundle By Name(w124) -> ("Global Rectangle"=w100:i32[])
            n37 = call "IMAQ IntegerToColorValue"("error in (no error)"=w66, "U32 value"=w120) -> ("error out"=w65:errorcluster, "Color Value"=w110:T49)  [unwired: 3 in, 2 out]
            n38 = Build Array(w120) -> (w111:u32[])
            n39 = call "IMAQ Overlay ROI"("Colors (Green)"=w111, "Group"=w85, "error in (no error)"=w89, "ROI Descriptor"=w124, "Image"=w91) -> ("error out"=w81:errorcluster, "Image Out"=w82:T1)  [unwired: 5 in]
            n40 = Index Array(array=w100) -> (element #1=w99:i32, element #2=w98:i32)  [unwired: 2 in]
            n41 = Merge Errors(w93, w101, w81, w65) -> (w109:errorcluster)
            n42 = call "Logical Processors Used.vi"() -> ("# Logical Processor Used"=w97:i32)  [unwired: 6 in]
            n43 = Select(t=w92, s=w125, f="Phasor Plot ROIs Overlay" ("Group")) -> (s? t:f=w95:string)
            n44 = for "For Loop on V Lines" {
              tunnel: w122 -> [w159] mode=indexing
              tunnel: w103 -> [w157]
              tunnel: w112 -> [w156]
              tunnel: w99 -> [w155]
              tunnel: w98 -> [w154]
              tunnel: w45 -> [w153]
              tunnel: w110 -> [w152]
              tunnel: w95 -> [w151]
              tunnel: [w148] -> w108
              tunnel: [w147] -> w106 mode=concatenating
              tunnel: w109 -> [w150]
              tunnel: [w149] -> w107
              tunnel: w94 -> [w146]
              tunnel: w123 -> [w145] mode=indexing
              workers-P: w97 -> [_]
              tunnel: w54 -> [w144]
              tunnel: w102 -> [w143]
              tunnel: w46 -> [w142]
              tunnel: w70 -> [w141]
              tunnel: w69 -> [w140]
              tunnel: w47 -> [w139]
              tunnel: w44 -> [w138]
              i -> [w158]
              # "y"
              n45 = for "For Loop on H columns" {
                tunnel: w159 -> [w183] mode=indexing
                tunnel: w158 -> [w177]
                tunnel: w157 -> [w182]
                tunnel: w156 -> [w181]
                tunnel: w155 -> [w180]
                tunnel: w154 -> [w179]
                tunnel: w153 -> [w178]
                tunnel: w152 -> [w175]
                tunnel: w151 -> [w174]
                tunnel: [w173] -> w148
                tunnel: w144 -> [w172]
                tunnel: [w171] -> w147 mode=indexing if=w167
                tunnel: w150 -> [w168]
                tunnel: [w170] -> w149
                tunnel: w146 -> [w169]
                tunnel: w145 -> [w166] mode=indexing
                tunnel: w143 -> [w165]
                tunnel: w142 -> [w164]
                tunnel: w141 -> [w163]
                tunnel: w140 -> [w162]
                tunnel: w139 -> [w161]
                tunnel: w138 -> [w160]
                i -> [w176]
                # "x"
                n46 = case shown="True" w166 {
                  tunnel: w183 -> [_ w213]
                  tunnel: w182 -> [_ _]
                  tunnel: w181 -> [_ w211]
                  tunnel: w180 -> [_ w207]
                  tunnel: w179 -> [_ w206]
                  tunnel: w178 -> [_ w205]
                  tunnel: w177 -> [_ w193]
                  tunnel: w176 -> [_ w194]
                  tunnel: w175 -> [_ w204]
                  tunnel: w174 -> [_ w203]
                  tunnel: [w185 w201] -> w173
                  tunnel: w172 -> [_ w199]
                  tunnel: [_ w190] -> w171
                  tunnel: [w184 w198] -> w170
                  tunnel: w169 -> [w185 w197]
                  tunnel: w168 -> [w184 w196]
                  tunnel: [_ w195] -> w167
                  tunnel: w165 -> [_ w192]
                  tunnel: w164 -> [_ w191]
                  tunnel: w163 -> [_ w189]
                  tunnel: w162 -> [_ w188]
                  tunnel: w161 -> [_ w187]
                  tunnel: w160 -> [_ w186]
                  frame False {
                  }
                  frame True {
                    n47 = Complex To Re/Im(x + iy=w213) -> (x=w214:sgl, y=w212:sgl)
                    n48 = call "AlliGator Convert Phasor Value to Phasor Image Coordinates (1).vim"("Phasor Plot Reference Points"=w211, "Phasor s"=w212, "Phasor g"=w214) -> ("Phasor Plot y"=w216:dbl, "Phasor Plot x"=w209:dbl)  [unwired: 7 in]
                    n49 = Compound Arithmetic op=ADD(invert w207, w209) -> (w210:dbl)
                    n50 = Compound Arithmetic op=ADD(w216, invert w206) -> (w208:dbl)
                    n51 = Bundle(w194, w193) -> (w190:cluster{i32, i32})  [unwired: 1 in]
                    n52 = Index Array(array=w192, index (row)=w208, index (col)=w210) -> (element=w215:u8)
                    n53 = Not Equal To 0?(x=w215) -> (x != 0?=w195:bool)
                    n54 = Compound Arithmetic op=AND(w199, w195) -> (w200:bool)
                    n55 = case shown="True" w200 {
                      tunnel: w205 -> [_ _]
                      tunnel: w193 -> [_ w229]
                      tunnel: w194 -> [_ w230]
                      tunnel: w204 -> [_ w220]
                      tunnel: w190 -> [_ w235]
                      tunnel: w203 -> [_ w234]
                      tunnel: w196 -> [w218 w224]
                      tunnel: [w218 w233] -> w202
                      tunnel: [w217 w232] -> w201
                      tunnel: w197 -> [w217 w231]
                      tunnel: w191 -> [_ w228]
                      tunnel: w189 -> [_ w221]
                      tunnel: w188 -> [_ w222]
                      tunnel: w187 -> [_ w219]
                      tunnel: w186 -> [_ w223]
                      frame False {
                        # "do not use image brightness"
                      }
                      frame True {
                        n56 = Index Array(array=w228, index (row)=w229, index (col)=w230) -> (element=w225:sgl)
                        n57 = call "Blend Overlay Color with Background.vi"("Overlay Color Value"=w220, "Image Scale Factor"=w222, "Blend Overlay with Background"=w219, "error in (no error)"=w224, "Image Display Range"=w223, "Image Color Array"=w221, "Pixel Value"=w225) -> ("error out"=w227:errorcluster, "Scaled/Blended Overlay Color Value"=w226:T49)  [unwired: 3 in]
                        n58 = call "IMAQ ColorValueToInteger"("error in (no error)"=w227, "Color Value"=w226) -> ("error out"=w237:errorcluster, "U32 value"=w236:u32)  [unwired: 3 in, 2 out]
                        n59 = call "IMAQ Overlay Points"("Color"=w236, "Group"=w234, "error in (no error)"=w237, "Point"=w235, "Image"=w231) -> ("error out"=w233:errorcluster, "Image Out"=w232:T1)  [unwired: 5 in]
                      }
                    }
                    n60 = call "Tiny Clear Error.vi"("Error In"=w202) -> ("no Error Out"=w198:errorcluster)  [unwired: 8 in]
                  }
                }
              }
            }
            n61 = case shown="False" w54 {
              tunnel: w108 -> [w135 w137]
              tunnel: [w133 w137] -> w80
              tunnel: w95 -> [w134 _]
              tunnel: w107 -> [w132 w136]
              tunnel: [w131 w136] -> w64
              tunnel: w106 -> [w130 _]
              tunnel: w120 -> [w129 _]
              frame False {
                # "do not use image brightness"
                n62 = call "IMAQ Overlay Points"("Color"=w129, "Group"=w134, "error in (no error)"=w132, "Array of Points"=w130, "Image"=w135) -> ("error out"=w131:errorcluster, "Image Out"=w133:T1)  [unwired: 5 in]
              }
              frame True {
                # "already highlighted"
              }
            }
            n63 = call "AlliGator Phasor Plot Image ROI Storage [SGL] v3.vi"("Current Phasor Plot ROI Color"=w120, "Error In"=w64, "Current ROI Descriptor"=w124, "Default Name (\"ROI\")"="", "Action"=AlliGator_ROI_Manager_Actions."Update Current ROI Descriptor") -> ("Error Out"=w63:errorcluster)  [unwired: 1 in, 5 out]
            n64 = call <vilib>:"Clear Errors.vi"("error in (no error)"=w63, "specific error code to clear (0: all)"=w121) -> ("error out"=w128:errorcluster)  [unwired: 4 in, 1 out]
            n65 = in-place-dvr #1() -> (w40:refnum<data-value>, w38:errorcluster)  [unwired: 1 in]
          }
          n66 = Merge Errors(w38, w43) -> (w39:errorcluster)
          n67 = call "High Resolution Timing.vi"("relative seconds (NaN)"=w34) -> ("elapsed (relative) seconds"=w33:dbl)  [unwired: 16 in, 2 out]
        }
        frame True {
        }
      }
    }
    frame Error {
    }
  }
  "Error Out" <- w11
  "CPU (s)" <- w8
  "AlliGator IV DVR out" <- w12
  "Phasor Plot Image Out" <- w5
  "Source Image Display out" <- w3
